vi "SaveTemporary.vi"(8 "error in (no error)":errorcluster, 11 "ctl in":refnum<class "ctl.lvclass">) -> (0 "error out":errorcluster, 2 "Temporary Control":path, 3 "ctl out":refnum<class "ctl.lvclass">)   [LabVIEW 2012, in "ctl.lvclass"]
uses:
  ctl.lvclass
  ctl.lvclass/ctl.ctl
  _ResManager_v86/IDCloneResMgr.lvlib
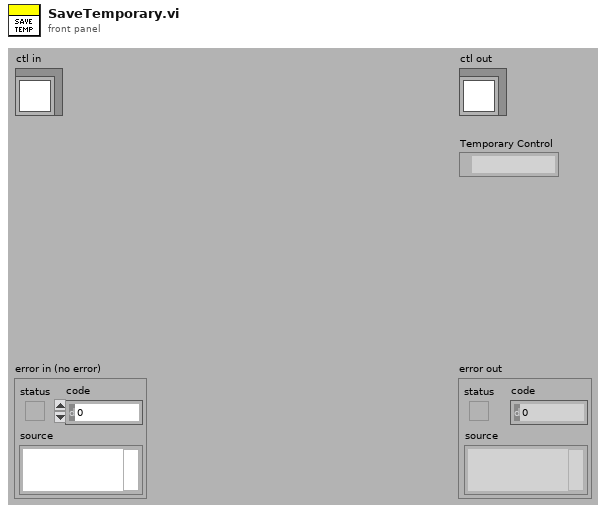
[diagram p1: front panel]
types:
  T1 = cluster{"type":u32, "id":i32, "name":string, "binary data":string}[]
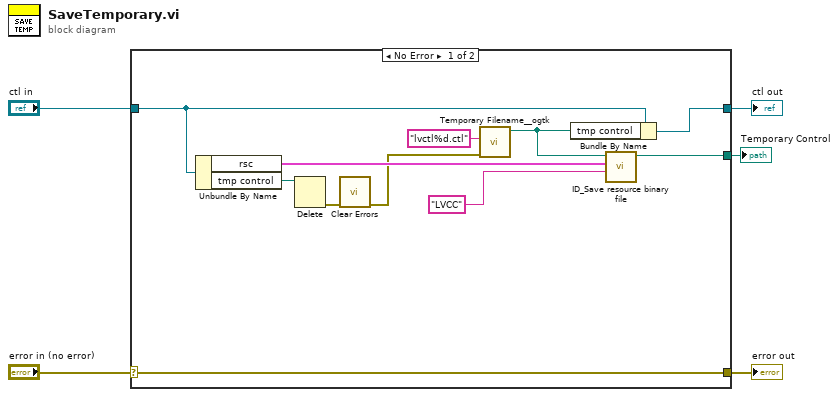
[diagram p0: block diagram]
diagram:
  n1 = case shown="No Error" "error in (no error)" {
    selector: "error in (no error)" -> [w15 w17]
    tunnel: [w15 w17] -> w4
    tunnel: [w11 w16] -> w2
    tunnel: "ctl in" -> [w12 w16]
    tunnel: [w7 _] -> w1
    frame No Error {
      n2 = Unbundle By Name(w12) -> ("rsc"=w14:T1, "tmp control"=w10:path)
      n3 = Delete(path (use dialog)=w10) -> (error out=w9:errorcluster)  [unwired: 4 in, 2 out]
      n4 = call <vilib>:"Clear Errors.vi"("error in (no error)"=w9) -> ("error out"=w8:errorcluster)  [unwired: 6 in]
      n5 = call <userlib>:"Temporary Filename__ogtk.vi"("error in (no error)"=w8, "pattern (lvtemp%d.tmp)"="lvctl%d.ctl") -> ("file in tmp dir"=w7:path)  [unwired: 4 in, 1 out]
      n6 = Bundle By Name(cluster=w12, "tmp control"=w7) -> (w11:refnum<class "ctl.lvclass">)
      n7 = call "ID_Save resource binary file.vi"("file type"="LVCC", "resources"=w14, "resource binary file"=w7) -> ()  [unwired: 9 out]
    }
    frame Error {
    }
  }
  "error out" <- w4
  "ctl out" <- w2
  "Temporary Control" <- w1
